vi "CRYSet Select Operator Window Configure.vi"(11 "Vi Ref":refnum<vi>) -> ()   [LabVIEW 2013]
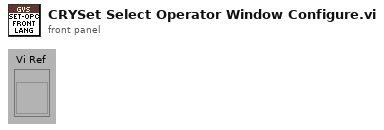
[diagram p1: front panel]
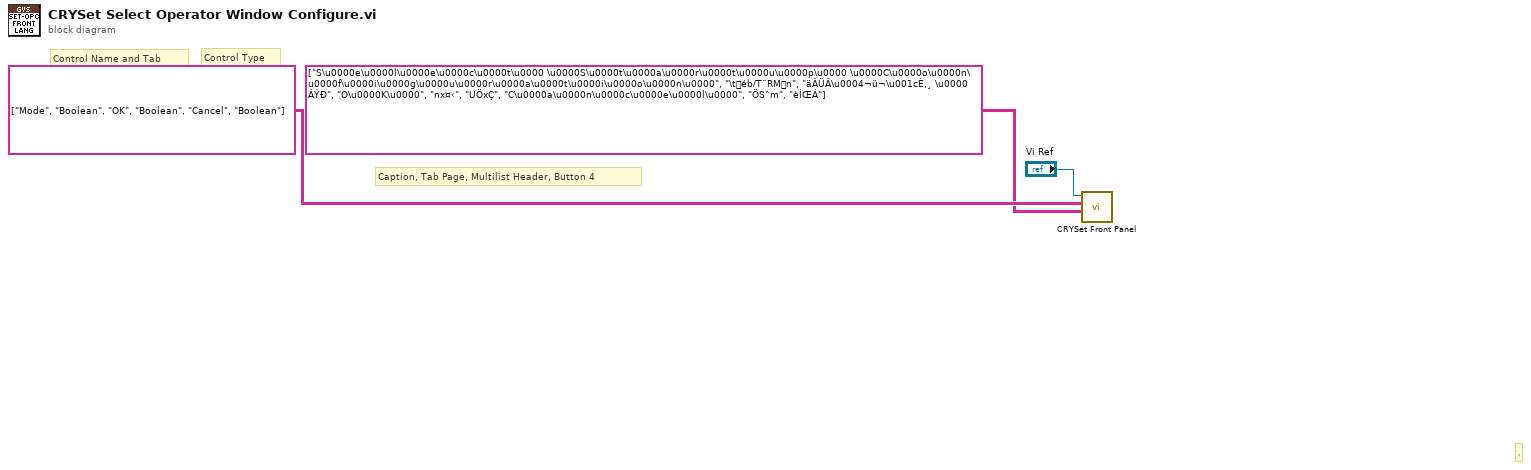
[diagram p0: block diagram]
diagram:
  # ","
  # "Caption, Tab Page, Multilist Header, Button 4"
  # "Control Type"
  # "Control Name and Tab"
  n1 = call "CRYSet Front Panel.vi"("Caption(Boolean Text)"=string[][] [["S\u0000e\u0000l\u0000e\u0000c\u0000t\u0000 \u0000S\u0000t\u0000a\u0000r\u0000t\u0000u\u0000p\u0000 \u0000C\u0000o\u0000n\u0000f\u0000i\u0000g\u0000u\u0000r\u0000a\u0000t\u0000i\u0000o\u0000n\u0000", "\téb/T¨RMn", "äÂÜÂ\u0004¬ü¬\u001cÈ,¸ \u0000 ÁÝÐ"], ["O\u0000K\u0000", "nx¤‹", "UÖxÇ"], ["C\u0000a\u0000n\u0000c\u0000e\u0000l\u0000", "ÖSˆm", "èÍŒÁ"]], "Control ID and Type(Label Name, Type)"=string[][] [["Mode", "Boolean"], ["OK", "Boolean"], ["Cancel", "Boolean"]], "Vi Ref"="Vi Ref") -> ()  [unwired: 9 in]
